vi "RubikTurnFSM.vi"() -> ()   [LabVIEW 2017]
uses:
  Projekt-RubikLibrary/ServoEnumControl.ctl
  Projekt-RubikLibrary/ServoAbsAngleControl_.ctl
  Projekt-RubikLibrary/ServoAbsAngleControl.ctl
  Projekt-RubikLibrary/RubikLibrary.lvlib
panel:
  in  "Servo":T1
  in  "Turn by":enum16{"-90°", "+90°"}(ring)
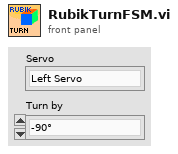
[diagram p1: front panel]
types:
  T1 = typedef "RubikLibrary.lvlib/ServoEnumControl.ctl" = enum16{"Left Servo", "Front Servo", "Right Servo"}
  T2 = typedef "ServoAbsAngleControl_.ctl" = enum16{"-90°", "0°", "+90°"}
  T3 = typedef "RubikLibrary.lvlib/ServoAbsAngleControl.ctl" = enum16{"-90°", "0°", "+90°"}
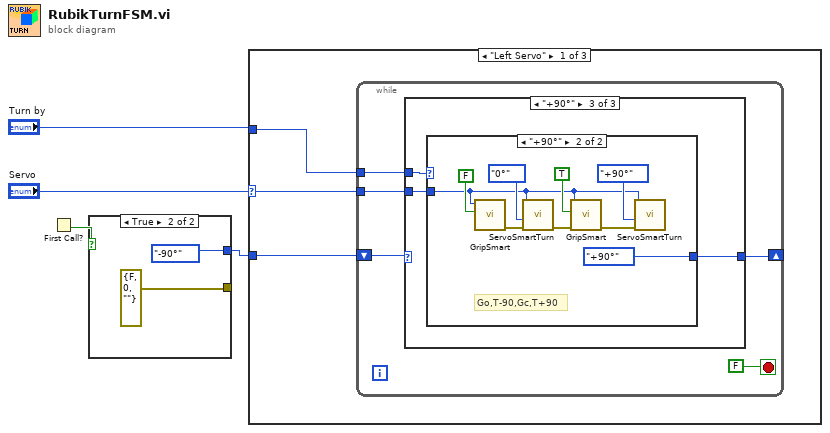
[diagram p0: block diagram]
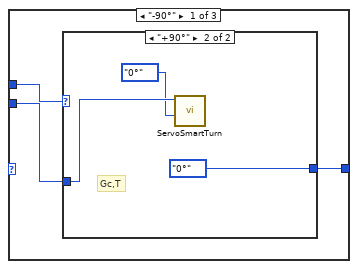
[diagram p3: hidden frame]
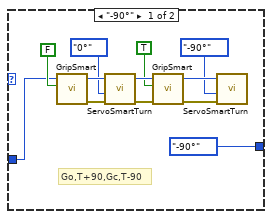
[diagram p4: hidden frame]
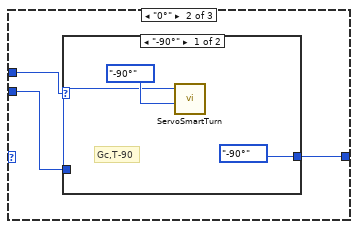
[diagram p5: hidden frame]
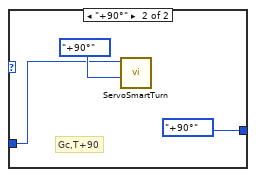
[diagram p6: hidden frame]
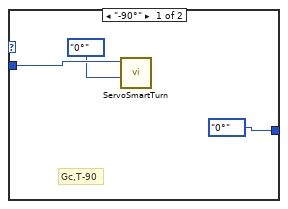
[diagram p7: hidden frame]
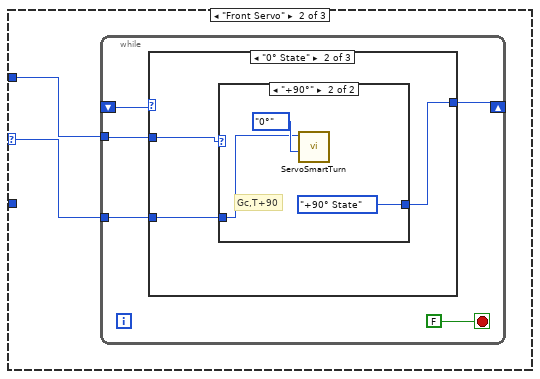
[diagram p8: hidden frame]
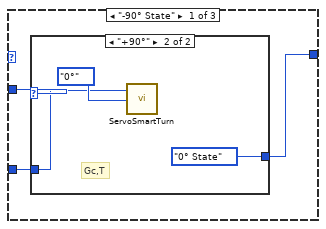
[diagram p9: hidden frame]
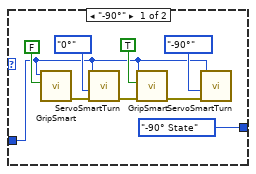
[diagram p10: hidden frame]
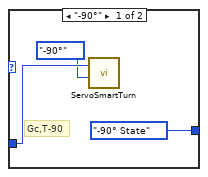
[diagram p11: hidden frame]
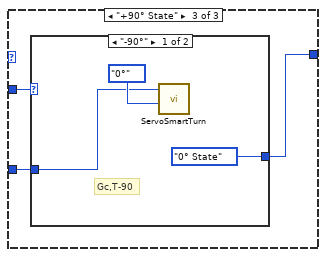
[diagram p12: hidden frame]
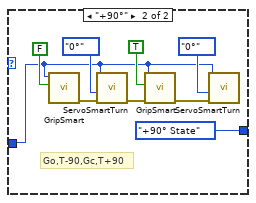
[diagram p13: hidden frame]
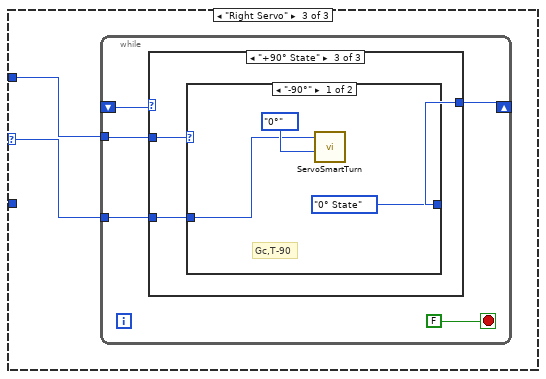
[diagram p14: hidden frame]
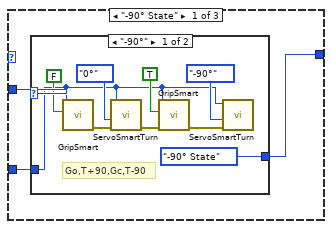
[diagram p15: hidden frame]
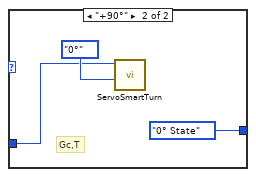
[diagram p16: hidden frame]
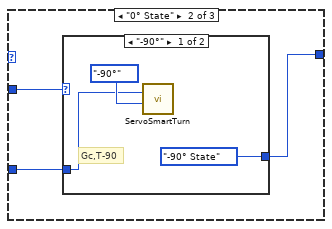
[diagram p17: hidden frame]
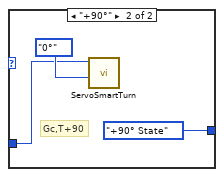
[diagram p18: hidden frame]
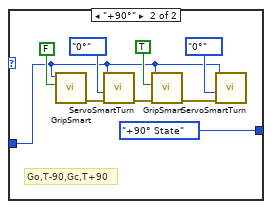
[diagram p19: hidden frame]
diagram:
  n1 = First Call?() -> (First Call?: T/F=w3:bool)
  n2 = case shown="True" w3 {
    tunnel: [_ errorcluster {"status"=FALSE, "code"=0, "source"=""} ("error in (no error)")] -> _
    tunnel: [_ ServoAbsAngleControl_."-90°" ("Turn to")] -> w2
    frame False {
    }
    frame True {
    }
  }
  n3 = case shown="\"Left Servo\"" "Servo" {
    selector: "Servo" -> [w8 w54 w100]
    tunnel: "Turn by" -> [w9 w55 w101]
    tunnel: w2 -> [w7 _ _]
    frame "Left Servo" {
      n4 = while {
        shift-right: [w14] -> _
        shift-left: w7 -> [w10]
        tunnel: w9 -> [w12]
        tunnel: w8 -> [w11]
        stop <- FALSE stop-if-true
        n5 = case shown="\"+90°\"" w10 {
          tunnel: [w17 w32 w41] -> w14
          tunnel: w12 -> [w16 w31 w40]
          tunnel: w11 -> [w15 w30 w39]
          frame "-90°" {
            n6 = case shown="\"+90°\"" w16 {
              tunnel: [ServoAbsAngleControl."-90°" ("Enum 2") ServoAbsAngleControl."0°" ("Enum 2")] -> w17
              tunnel: w15 -> [w21 w28]
              frame "-90°" {
                # "Go,T+90,Gc,T-90"
                n7 = call "GripSmart.vi"("Turn to (in)"=FALSE, "Servo"=w21) -> ("error out"=w24:errorcluster)  [unwired: 8 in, 1 out]
                n8 = call "ServoSmartTurn.vi"("error in"=w24, "Turn to (in)"=ServoAbsAngleControl."0°" ("Turn to"), "Servo"=w21) -> ("error out"=w23:errorcluster)  [unwired: 7 in, 1 out]
                n9 = call "GripSmart.vi"("error in"=w23, "Turn to (in)"=TRUE, "Servo"=w21) -> ("error out"=w22:errorcluster)  [unwired: 7 in, 1 out]
                n10 = call "ServoSmartTurn.vi"("error in"=w22, "Turn to (in)"=ServoAbsAngleControl."-90°" ("Turn to"), "Servo"=w21) -> ()  [unwired: 7 in, 2 out]
              }
              frame "+90°" {
                # "Gc,T"
                n11 = call "ServoSmartTurn.vi"("Turn to (in)"=ServoAbsAngleControl_."0°" ("Turn to"), "Servo"=w28) -> ()  [unwired: 8 in, 2 out]
              }
            }
          }
          frame "0°" {
            n12 = case shown="\"-90°\"" w31 {
              tunnel: [ServoAbsAngleControl."-90°" ("Enum 2") ServoAbsAngleControl."+90°" ("Enum 2")] -> w32
              tunnel: w30 -> [w33 w36]
              frame "-90°" {
                # "Gc,T-90"
                n13 = call "ServoSmartTurn.vi"("Turn to (in)"=ServoAbsAngleControl."-90°" ("Turn to"), "Servo"=w33) -> ()  [unwired: 8 in, 2 out]
              }
              frame "+90°" {
                # "Gc,T+90"
                n14 = call "ServoSmartTurn.vi"("Turn to (in)"=ServoAbsAngleControl."+90°" ("Turn to"), "Servo"=w36) -> ()  [unwired: 8 in, 2 out]
              }
            }
          }
          frame "+90°" {
            n15 = case shown="\"+90°\"" w40 {
              tunnel: [ServoAbsAngleControl."0°" ("Enum 2") ServoAbsAngleControl."+90°" ("Enum 2")] -> w41
              tunnel: w39 -> [w43 w45]
              frame "-90°" {
                # "Gc,T-90"
                n16 = call "ServoSmartTurn.vi"("Turn to (in)"=ServoAbsAngleControl."0°" ("Turn to"), "Servo"=w43) -> ()  [unwired: 8 in, 2 out]
              }
              frame "+90°" {
                # "Go,T-90,Gc,T+90"
                n17 = call "GripSmart.vi"("Turn to (in)"=FALSE, "Servo"=w45) -> ("error out"=w51:errorcluster)  [unwired: 8 in, 1 out]
                n18 = call "ServoSmartTurn.vi"("error in"=w51, "Turn to (in)"=ServoAbsAngleControl."0°" ("Turn to"), "Servo"=w45) -> ("error out"=w50:errorcluster)  [unwired: 7 in, 1 out]
                n19 = call "GripSmart.vi"("error in"=w50, "Turn to (in)"=TRUE, "Servo"=w45) -> ("error out"=w49:errorcluster)  [unwired: 7 in, 1 out]
                n20 = call "ServoSmartTurn.vi"("error in"=w49, "Turn to (in)"=ServoAbsAngleControl."+90°" ("Turn to"), "Servo"=w45) -> ()  [unwired: 7 in, 2 out]
              }
            }
          }
        }
      }
    }
    frame "Front Servo" {
      n21 = while {
        shift-right: [w59] -> _
        shift-left: _ -> [w60]
        tunnel: w55 -> [w57]
        tunnel: w54 -> [w56]
        stop <- FALSE stop-if-true
        n22 = case shown="\"0° State\"" w60 {
          tunnel: [w63 w78 w87] -> w59
          tunnel: w57 -> [w62 w77 w86]
          tunnel: w56 -> [w61 w76 w85]
          frame "-90° State" {
            n23 = case shown="\"+90°\"" w62 {
              tunnel: [enum16{"-90° State", "0° State", "+90° State"}."-90° State" ("Enum 2") enum16{"-90° State", "0° State", "+90° State"}."0° State" ("Enum 2")] -> w63
              tunnel: w61 -> [w64 w73]
              frame "-90°" {
                n24 = call "GripSmart.vi"("Turn to (in)"=FALSE, "Servo"=w64) -> ("error out"=w70:errorcluster)  [unwired: 8 in, 1 out]
                n25 = call "ServoSmartTurn.vi"("error in"=w70, "Turn to (in)"=ServoAbsAngleControl."0°" ("Turn to"), "Servo"=w64) -> ("error out"=w69:errorcluster)  [unwired: 7 in, 1 out]
                n26 = call "GripSmart.vi"("error in"=w69, "Turn to (in)"=TRUE, "Servo"=w64) -> ("error out"=w68:errorcluster)  [unwired: 7 in, 1 out]
                n27 = call "ServoSmartTurn.vi"("error in"=w68, "Turn to (in)"=ServoAbsAngleControl."-90°" ("Turn to"), "Servo"=w64) -> ()  [unwired: 7 in, 2 out]
              }
              frame "+90°" {
                # "Gc,T"
                n28 = call "ServoSmartTurn.vi"("Turn to (in)"=ServoAbsAngleControl."0°" ("Turn to"), "Servo"=w73) -> ()  [unwired: 8 in, 2 out]
              }
            }
          }
          frame "0° State" {
            n29 = case shown="\"+90°\"" w77 {
              tunnel: [enum16{"-90° State", "0° State", "+90° State"}."-90° State" ("Enum 2") enum16{"-90° State", "0° State", "+90° State"}."+90° State" ("Enum 2")] -> w78
              tunnel: w76 -> [w80 w82]
              frame "-90°" {
                # "Gc,T-90"
                n30 = call "ServoSmartTurn.vi"("Turn to (in)"=ServoAbsAngleControl."-90°" ("Turn to"), "Servo"=w80) -> ()  [unwired: 8 in, 2 out]
              }
              frame "+90°" {
                # "Gc,T+90"
                n31 = call "ServoSmartTurn.vi"("Turn to (in)"=ServoAbsAngleControl."0°" ("Turn to"), "Servo"=w82) -> ()  [unwired: 8 in, 2 out]
              }
            }
          }
          frame "+90° State" {
            n32 = case shown="\"-90°\"" w86 {
              tunnel: [enum16{"-90° State", "0° State", "+90° State"}."0° State" ("Enum 2") enum16{"-90° State", "0° State", "+90° State"}."+90° State" ("Enum 2")] -> w87
              tunnel: w85 -> [w88 w91]
              frame "-90°" {
                # "Gc,T-90"
                n33 = call "ServoSmartTurn.vi"("Turn to (in)"=ServoAbsAngleControl."0°" ("Turn to"), "Servo"=w88) -> ()  [unwired: 8 in, 2 out]
              }
              frame "+90°" {
                # "Go,T-90,Gc,T+90"
                n34 = call "GripSmart.vi"("Turn to (in)"=FALSE, "Servo"=w91) -> ("error out"=w97:errorcluster)  [unwired: 8 in, 1 out]
                n35 = call "ServoSmartTurn.vi"("error in"=w97, "Turn to (in)"=ServoAbsAngleControl."0°" ("Turn to"), "Servo"=w91) -> ("error out"=w96:errorcluster)  [unwired: 7 in, 1 out]
                n36 = call "GripSmart.vi"("error in"=w96, "Turn to (in)"=TRUE, "Servo"=w91) -> ("error out"=w95:errorcluster)  [unwired: 7 in, 1 out]
                n37 = call "ServoSmartTurn.vi"("error in"=w95, "Turn to (in)"=ServoAbsAngleControl."0°" ("Turn to"), "Servo"=w91) -> ()  [unwired: 7 in, 2 out]
              }
            }
          }
        }
      }
    }
    frame "Right Servo" {
      n38 = while {
        shift-right: [w105] -> _
        shift-left: _ -> [w106]
        tunnel: w101 -> [w103]
        tunnel: w100 -> [w102]
        stop <- FALSE stop-if-true
        n39 = case shown="\"+90° State\"" w106 {
          tunnel: [w109 w124 w133] -> w105
          tunnel: w103 -> [w108 w123 w132]
          tunnel: w102 -> [w107 w122 w131]
          frame "-90° State" {
            n40 = case shown="\"-90°\"" w108 {
              tunnel: [enum16{"-90° State", "0° State", "+90° State"}."-90° State" ("Enum 2") enum16{"-90° State", "0° State", "+90° State"}."0° State" ("Enum 2")] -> w109
              tunnel: w107 -> [w110 w119]
              frame "-90°" {
                # "Go,T+90,Gc,T-90"
                n41 = call "GripSmart.vi"("Turn to (in)"=FALSE, "Servo"=w110) -> ("error out"=w116:errorcluster)  [unwired: 8 in, 1 out]
                n42 = call "ServoSmartTurn.vi"("error in"=w116, "Turn to (in)"=ServoAbsAngleControl."0°" ("Turn to"), "Servo"=w110) -> ("error out"=w115:errorcluster)  [unwired: 7 in, 1 out]
                n43 = call "GripSmart.vi"("error in"=w115, "Turn to (in)"=TRUE, "Servo"=w110) -> ("error out"=w114:errorcluster)  [unwired: 7 in, 1 out]
                n44 = call "ServoSmartTurn.vi"("error in"=w114, "Turn to (in)"=ServoAbsAngleControl."-90°" ("Turn to"), "Servo"=w110) -> ()  [unwired: 7 in, 2 out]
              }
              frame "+90°" {
                # "Gc,T"
                n45 = call "ServoSmartTurn.vi"("Turn to (in)"=ServoAbsAngleControl."0°" ("Turn to"), "Servo"=w119) -> ()  [unwired: 8 in, 2 out]
              }
            }
          }
          frame "0° State" {
            n46 = case shown="\"-90°\"" w123 {
              tunnel: [enum16{"-90° State", "0° State", "+90° State"}."-90° State" ("Enum 2") enum16{"-90° State", "0° State", "+90° State"}."+90° State" ("Enum 2")] -> w124
              tunnel: w122 -> [w125 w128]
              frame "-90°" {
                # "Gc,T-90"
                n47 = call "ServoSmartTurn.vi"("Turn to (in)"=ServoAbsAngleControl."-90°" ("Turn to"), "Servo"=w125) -> ()  [unwired: 8 in, 2 out]
              }
              frame "+90°" {
                # "Gc,T+90"
                n48 = call "ServoSmartTurn.vi"("Turn to (in)"=ServoAbsAngleControl."0°" ("Turn to"), "Servo"=w128) -> ()  [unwired: 8 in, 2 out]
              }
            }
          }
          frame "+90° State" {
            n49 = case shown="\"-90°\"" w132 {
              tunnel: [enum16{"-90° State", "0° State", "+90° State"}."0° State" ("Enum 2") enum16{"-90° State", "0° State", "+90° State"}."+90° State" ("Enum 2")] -> w133
              tunnel: w131 -> [w134 w137]
              frame "-90°" {
                # "Gc,T-90"
                n50 = call "ServoSmartTurn.vi"("Turn to (in)"=ServoAbsAngleControl."0°" ("Turn to"), "Servo"=w134) -> ()  [unwired: 8 in, 2 out]
              }
              frame "+90°" {
                # "Go,T-90,Gc,T+90"
                n51 = call "GripSmart.vi"("Turn to (in)"=FALSE, "Servo"=w137) -> ("error out"=w143:errorcluster)  [unwired: 8 in, 1 out]
                n52 = call "ServoSmartTurn.vi"("error in"=w143, "Turn to (in)"=ServoAbsAngleControl."0°" ("Turn to"), "Servo"=w137) -> ("error out"=w142:errorcluster)  [unwired: 7 in, 1 out]
                n53 = call "GripSmart.vi"("error in"=w142, "Turn to (in)"=TRUE, "Servo"=w137) -> ("error out"=w141:errorcluster)  [unwired: 7 in, 1 out]
                n54 = call "ServoSmartTurn.vi"("error in"=w141, "Turn to (in)"=ServoAbsAngleControl."0°" ("Turn to"), "Servo"=w137) -> ()  [unwired: 7 in, 2 out]
              }
            }
          }
        }
      }
    }
  }
